vi "Call Printer.vi"(0 "VISA资源名称":refnum<visa-resource-name>="COM2", 1 "IP":string, 2 "Data in":string, 3 "Error in":errorcluster caption="错误输入（无错误）", 4 "Use TCP?":bool) -> (5 "Data out":string, 6 "error out":errorcluster)   [LabVIEW 2014]
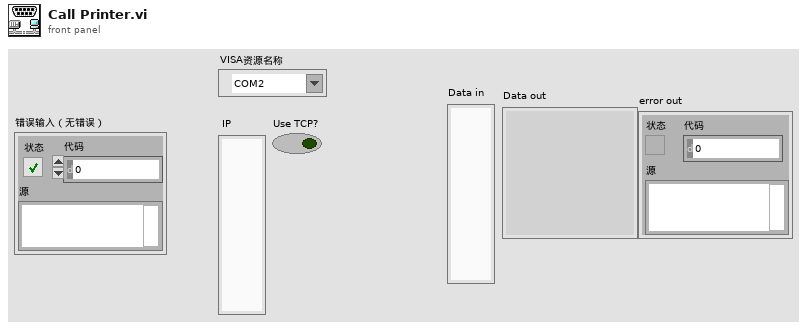
[diagram p1: front panel]
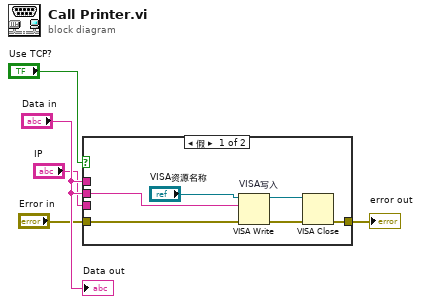
[diagram p0: block diagram]
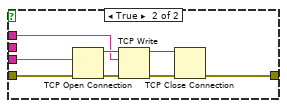
[diagram p2: hidden frame]
diagram:
  n1 = case shown="假" "Use TCP?" {
    tunnel: [w11 w14] -> w5
    tunnel: "Data in" -> [w7 _]
    tunnel: "Data in" -> [_ w17]
    tunnel: "IP" -> [_ w13]
    tunnel: "Error in" -> [w6 w12]
    frame False {
      n2 = VISA Write "VISA写入"(VISA resource name="VISA资源名称", write buffer=w7, error in (no error)=w6) -> (VISA resource name out=w9:refnum<visa-resource-name>, error out=w8:errorcluster)  [unwired: 1 out]
      n3 = VISA Close(VISA resource name=w9, error in (no error)=w8) -> (error out=w11:errorcluster)
    }
    frame True {
      n4 = TCP Open Connection(remote port or service name=w13, error in (no error)=w12) -> (connection ID=w18:refnum<k5>, error out=w19:errorcluster)  [unwired: 3 in]
      n5 = TCP Write(connection ID=w18, data in=w17, error in (no error)=w19) -> (connection ID out=w16:refnum<k5>, error out=w15:errorcluster)  [unwired: 1 in, 1 out]
      n6 = TCP Close Connection(connection ID=w16, error in (no error)=w15) -> (error out=w14:errorcluster)  [unwired: 1 in, 1 out]
    }
  }
  "error out" <- w5
  "Data out" <- "Data in"
